vi "pairwise method.vi"() -> ()   [LabVIEW 2014]
uses:
  <vilib>/Analysis/NI_AALBase.lvlib
panel:
  out "Histogram Graph":T1(graph)
  out "Waveform Graph":dbl[](graph)
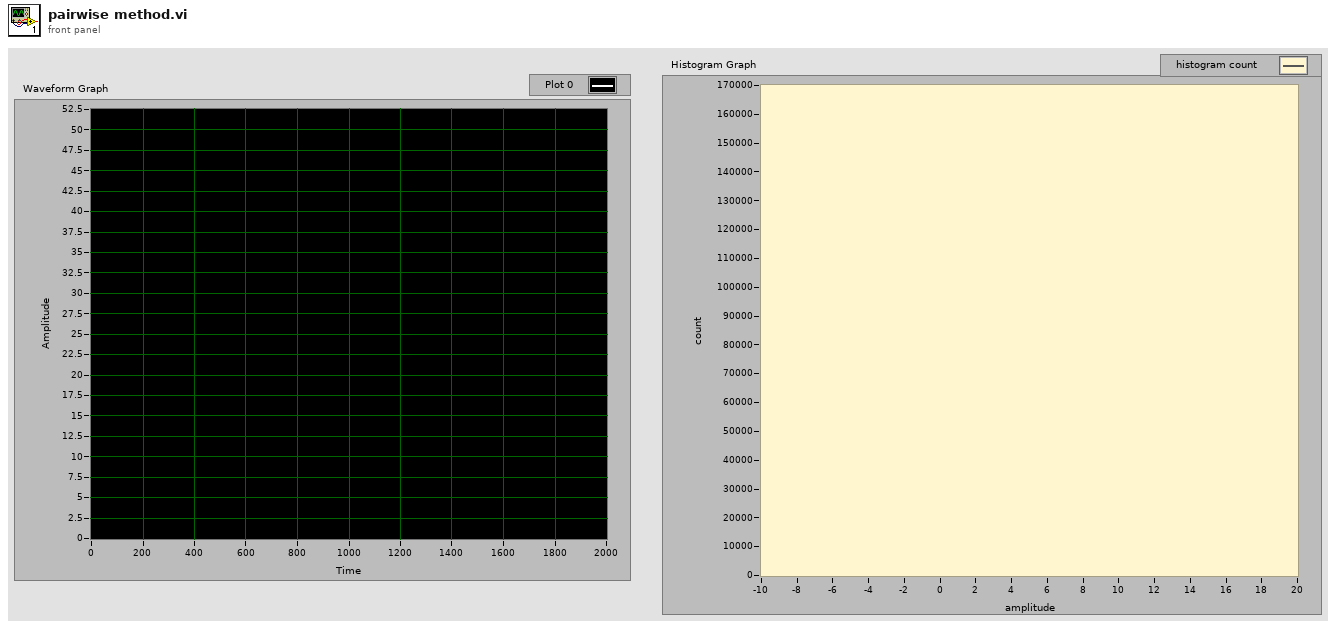
[diagram p1: front panel]
types:
  T1 = cluster{"X Values":dbl[], "Histogram: h(x)":i32[]}
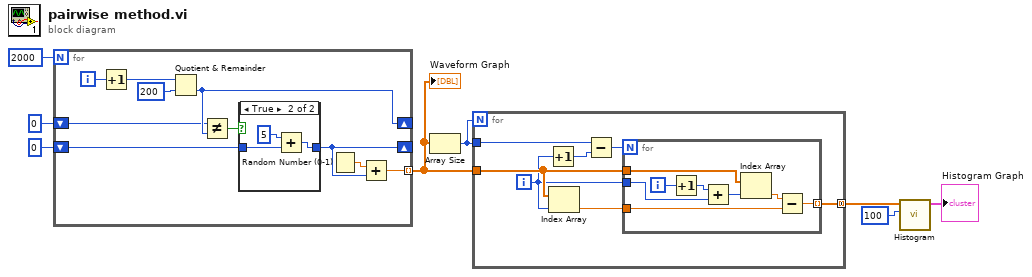
[diagram p0: block diagram]
diagram:
  n1 = for {
    N: 2000 -> [_]
    shift-right: [w14] -> _
    shift-left: 0 -> [w13]
    shift-right: [w11] -> _
    shift-left: 0 -> [w12]
    tunnel: [w9] -> w5 mode=indexing
    i -> [w16]
    n2 = Increment(x=w16) -> (x+1=w15:i32)
    n3 = Quotient & Remainder(x=w15, y=200) -> (floor(x/y)=w14:i32)  [unwired: 1 out]
    n4 = Not Equal?(x=w13, y=w14) -> (x != y?=w10:bool)
    n5 = case shown="True" w10 {
      tunnel: w12 -> [w19 w22]
      tunnel: [w19 w20] -> w11
      frame False {
      }
      frame True {
        n6 = Add(x=5, y=w22) -> (x+y=w20:i32)
      }
    }
    n7 = Random Number (0-1)() -> (number: 0 to 1=w18:dbl)
    n8 = Add(x=w18, y=w11) -> (x+y=w9:dbl)
  }
  "Waveform Graph" <- w5
  n9 = Array Size(array=w5) -> (size(s)=w4:i32)
  n10 = for {
    N: w4 -> [_]
    tunnel: w5 -> [w27]
    tunnel: [w28] -> w3 mode=concatenating
    tunnel: w4 -> [w25]
    i -> [w23]
    n11 = Increment(x=w23) -> (x+1=w24:i32)
    n12 = Index Array(array=w27, index=w23) -> (element=w29:dbl)
    n13 = Subtract(x=w25, y=w24) -> (x-y=w26:i32)
    n14 = for {
      N: w26 -> [_]
      tunnel: w29 -> [w34]
      tunnel: w27 -> [w37]
      tunnel: [w33] -> w28 mode=indexing
      tunnel: w23 -> [w31]
      i -> [w36]
      n15 = Increment(x=w36) -> (x+1=w32:i32)
      n16 = Add(x=w32, y=w31) -> (x+y=w30:i32)
      n17 = Index Array(array=w37, index=w30) -> (element=w35:dbl)
      n18 = Subtract(x=w35, y=w34) -> (x-y=w33:dbl)
    }
  }
  n19 = call <vilib>:"Histogram.vi"("intervals"=100, "X"=w3) -> ("Histogram Graph"=→"Histogram Graph":T1)  [unwired: 6 in, 3 out]
